vi "moving_average.vi"() -> ()   [LabVIEW 2012]
doc: "Moving average,\n\nThis program calculates and displays the moving average, with a pre-selected number. First of all, the program initialized two shift registers. The top shift register is initialized with one element and this register continiously adds the previous value with the new value. This shift register keeps the total of the last xx measurements. When dividing the results of the add function with the pre-selected value, we can calculate the moving average value. The bottom shift register contains an array with the dimension \"Average\". This shift register keeps all values of the measurement. The replacement function replaces every loop the new value. \n \nThis method is very efficent and fast, because we using the replace element function inside the loop and before we enter the while loop we initialzes the array. This VI was created in LabVIEW 6.1."
panel:
  in  "stop":bool
  out "?":cluster{dbl, dbl}(graph)
  in  "Average":i32=25
  # "Select the moving average and then\nrun the VI.  The chart will show the\ncurrent measurement and the \nresulting moving average."
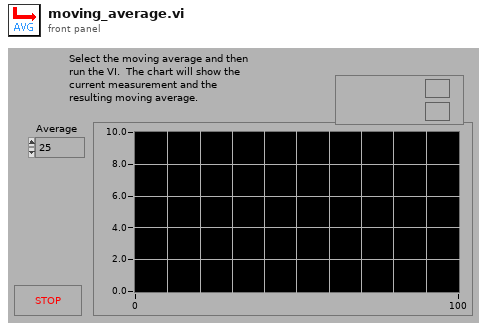
[diagram p1: front panel]
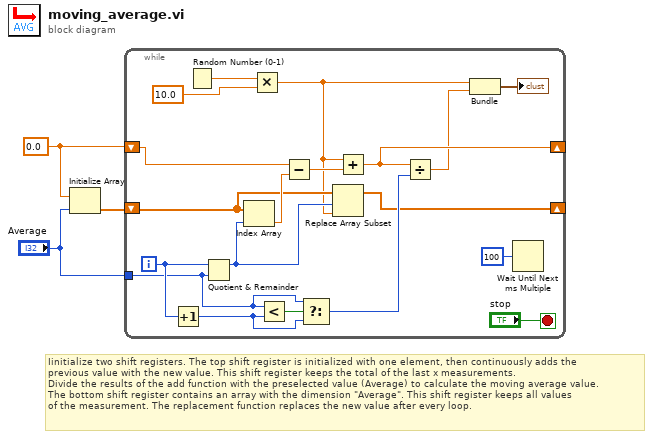
[diagram p0: block diagram]
diagram:
  w1 = 0.0 ("y")
  # "Iinitialize two shift registers. The top shift register is initialized with one element, then continuously adds the \nprevious value with the new value. This shift register keeps the total of the last x measurements. \nDivide the results of the add function with the preselected value (Average) to calculate the moving average value.\nThe bottom shift register contains an array with the dimension \"Average\". This shift register keeps all values \nof the measurement. The replacement function replaces the new value after every loop."
  n1 = Initialize Array(w1, "Average") -> (w3:dbl[])
  n2 = while {
    tunnel: "Average" -> [w5]
    shift-left: w3 -> [w20]
    shift-right: [w4] -> _
    shift-left: w1 -> [w18]
    shift-right: [w16] -> _
    i -> [w11]
    stop <- "stop" stop-if-true
    n3 = Increment(x=w11) -> (x+1=w8:i32)
    n4 = Random Number (0-1)() -> (number: 0 to 1=w7:dbl)
    n5 = Quotient & Remainder(x=w11, y=w5) -> (x-y*floor(x/y)=w17:i32)  [unwired: 1 out]
    n6 = Index Array(array=w20, index=w17) -> (element=w21:dbl)
    n7 = Multiply(x=w7, y=10.0) -> (x*y=w15:dbl)
    n8 = Less?(x=w5, y=w8) -> (x < y?=w10:bool)
    n9 = Subtract(x=w18, y=w21) -> (x-y=w19:dbl)
    n10 = Select(t=w5, s=w10, f=w8) -> (s? t:f=w9:i32)
    n11 = Replace Array Subset(array=w20, new element=w15, index=w17) -> (w4:dbl[])
    n12 = Add(x=w15, y=w19) -> (x+y=w16:dbl)
    n13 = Divide(x=w16, y=w9) -> (x/y=w14:dbl)
    n14 = Bundle(w15, w14) -> (→"?":cluster{dbl, dbl})  [unwired: 1 in]
    n15 = Wait Until Next ms Multiple(millisecond multiple=u32 100) -> ()  [unwired: 1 out]
  }
